vi "UserTable.vi"(8 "error in (no error)":errorcluster, 11 "MemberTable.lvclass":refnum<class "MemberTable.lvclass">) -> (0 "error out":errorcluster, 3 "MemberTable.lvclass":refnum<class "MemberTable.lvclass">)   [LabVIEW 2015, in "Member_Actor.lvlib"]
uses:
  Member_Actor.lvlib
  MemberTable/MemberTable.lvclass
  <vilib>/Utility/error.llb/Error Cluster From Error Code.vi
  <vilib>/ErrorRing/Error Ring.xnode
panel:
  in  "修改课程表":bool
  in  "课程表":cluster{"结束周":dbl, "起始周":dbl, "课程名称":string}[][](array[cluster])
  in  "Stop":bool
  # "—"
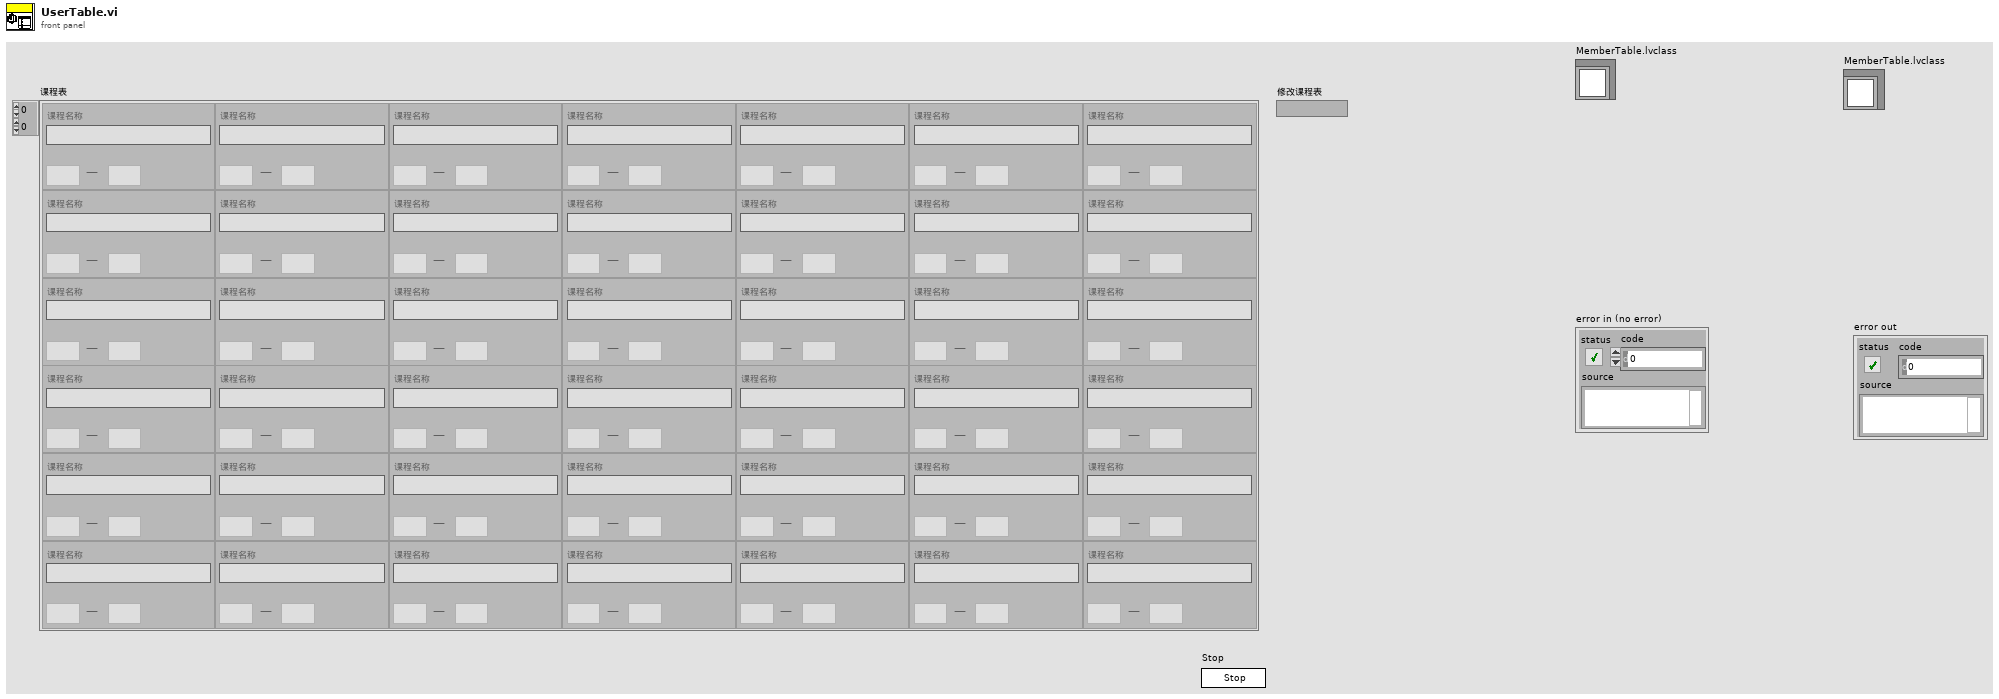
[diagram p1: front panel]
types:
  T1 = enum32{"Invalid", "Standard", "Closed", "Hidden", "Minimized", "Maximized"}
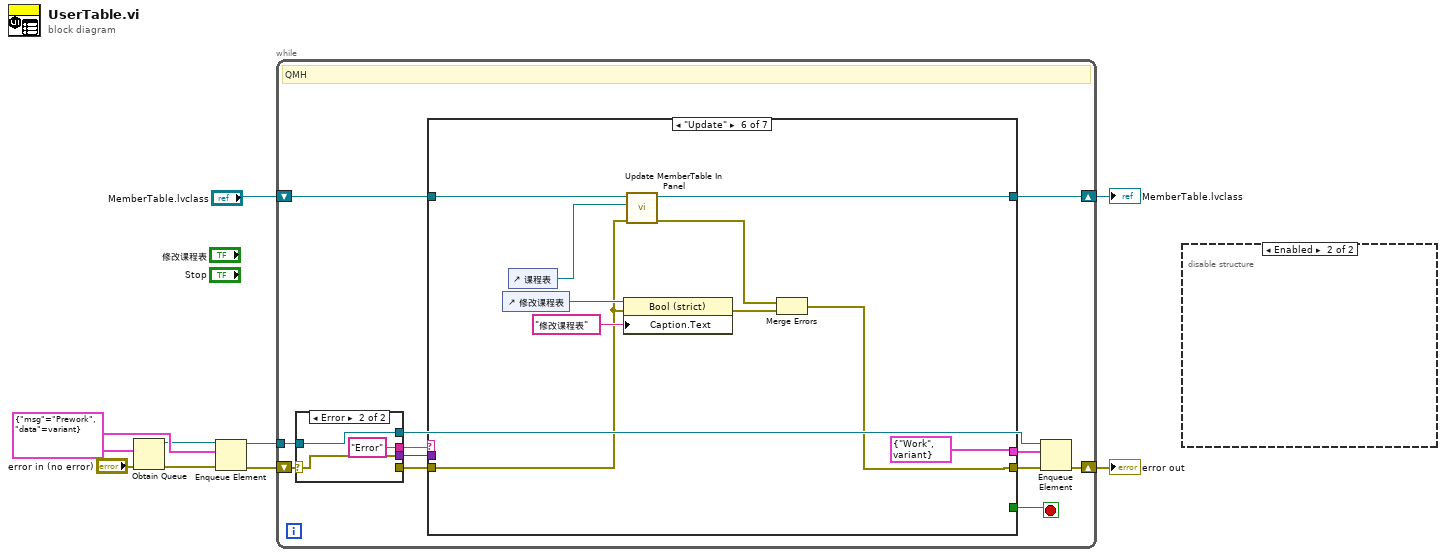
[diagram p0: block diagram]
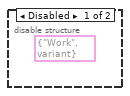
[diagram p2: hidden frame]
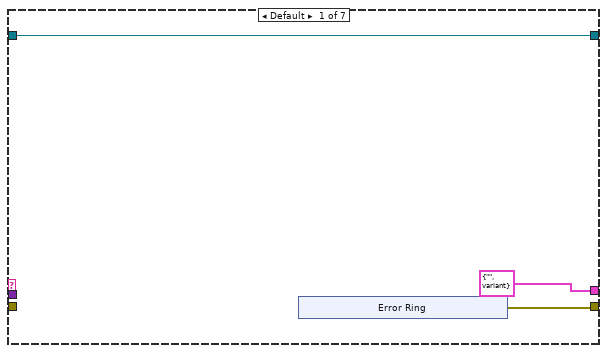
[diagram p3: hidden frame]
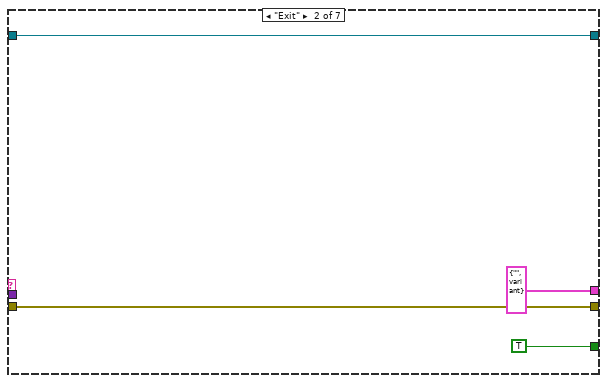
[diagram p4: hidden frame]
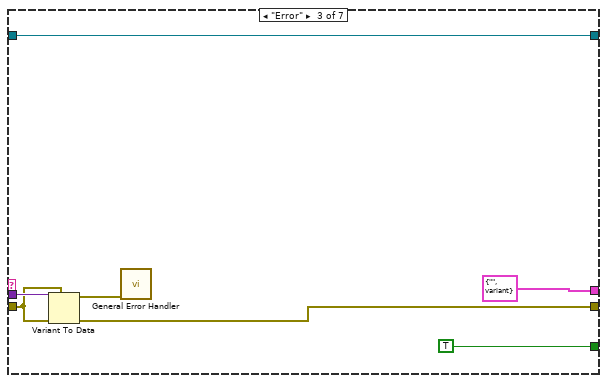
[diagram p5: hidden frame]
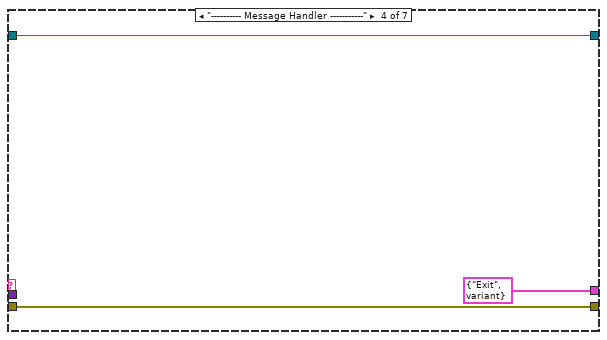
[diagram p6: hidden frame]
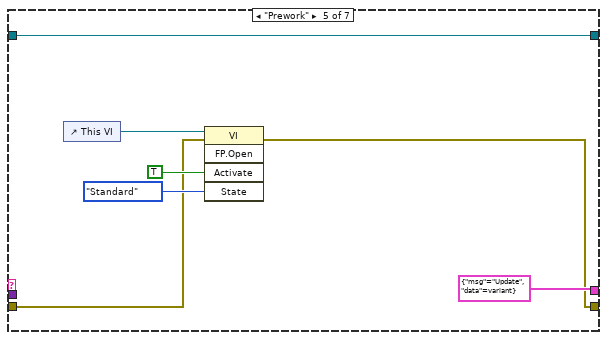
[diagram p7: hidden frame]
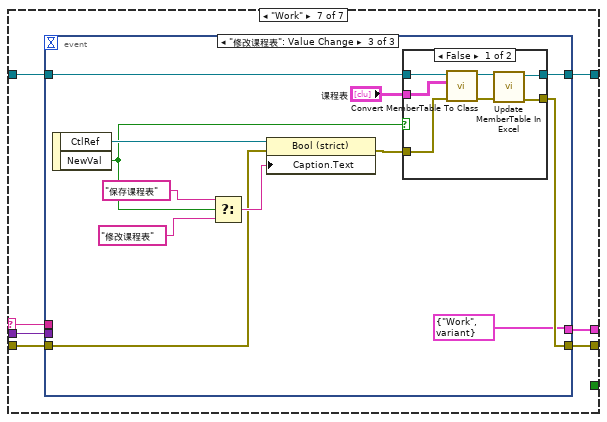
[diagram p8: hidden frame]
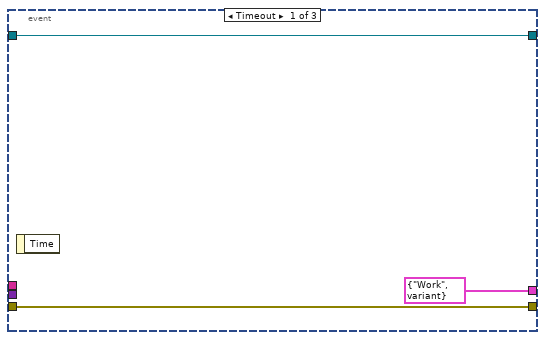
[diagram p9: hidden frame]
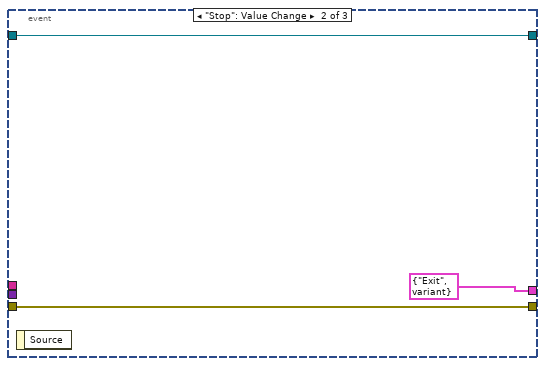
[diagram p10: hidden frame]
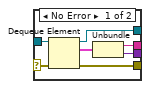
[diagram p12: hidden frame]
diagram:
  w7 = cluster{"msg":string, "data":variant} {"msg"="Prework", "data"=variant}
  n1 = Obtain Queue(element data type=w7, error in (no error)="error in (no error)") -> (queue out=w5:refnum<queue>, error out=w6:errorcluster)  [unwired: 3 in, 1 out]
  n2 = Enqueue Element(queue=w5, element=w7, error in (no error)=w6) -> (queue out=w8:refnum<queue>, error out=w9:errorcluster)  [unwired: 1 in, 1 out]
  n3 = while {
    tunnel: w8 -> [w20]
    shift-right: [w15] -> w2
    shift-left: w9 -> [w21]
    shift-right: [w10] -> w3
    shift-left: "MemberTable.lvclass" -> [w11]
    stop <- w12 stop-if-true
    # "QMH"
    n4 = case shown="Error" w21 {
      selector: w21 -> [w100 w104]
      tunnel: w20 -> [w101 w102]
      tunnel: [w99 _] -> w19
      tunnel: [w97 "Error" ("msg")] -> w18
      tunnel: [w96 w104] -> w17
      tunnel: [w95 w102] -> w14
      frame No Error {
        n5 = Dequeue Element(queue=w101, error in (no error)=w100) -> (queue out=w95:refnum<queue>, element=w98:cluster{"msg":string, "data":variant}, error out=w99:errorcluster)  [unwired: 1 in, 1 out]
        n6 = Unbundle(w98) -> ("msg"=w97:string, "data"=w96:variant)
      }
      frame Error {
      }
    }
    n7 = case shown="\"Update\"" w18 {
      selector: w18 -> [_ _ _ _ _ _ w65]
      tunnel: w19 -> [_ w33 w39 w43 w45 w55 w67]
      tunnel: w17 -> [_ _ w40 _ _ _ w66]
      tunnel: [w24 w33 w37 w43 w44 w52 w64] -> w16
      tunnel: [cluster{"msg":string, "data":variant} {"msg"="", "data"=variant} cluster{"msg":string, "data":variant} {"msg"="", "data"=variant} cluster{"msg":string, "data":variant} {"msg"="", "data"=variant} cluster{"msg":string, "data":variant} {"msg"="Exit", "data"=variant} cluster{"msg":string, "data":variant} {"msg"="Update", "data"=variant} cluster{"msg":string, "data":variant} {"msg"="Work", "data"=variant} w63] -> w13
      tunnel: [_ TRUE TRUE _ _ _ _] -> w12
      tunnel: w11 -> [w22 w30 w34 w41 w49 w59 w62]
      tunnel: [w22 w30 w34 w41 w49 w51 w61] -> w10
      frame Default {
        n8 = xnode "Error Ring"() -> ("error out"=w24:errorcluster)
      }
      frame "Exit" {
      }
      frame "Error" {
        n9 = Variant To Data(error in=w39, type=w39, Variant=w40) -> (data=w38:errorcluster, error out=w37:errorcluster)
        n10 = call <vilib>:"General Error Handler.vi"("error in (no error)"=w38) -> ()  [unwired: 10 in, 5 out]
      }
      frame "---------- Message Handler -----------" {
      }
      frame "Prework" {
        n11 = control-ref of="This VI"() -> (w48:refnum<vi>)
        n12 = invoke class="VI" method="FP.Open"(reference=w48, error in=w45, "Activate"=TRUE ("Activate?"), "State"=T1."Standard") -> (error out=w44:errorcluster)  [unwired: 1 in, 4 out]
      }
      frame "Update" {
        n13 = control-ref of="修改课程表"() -> (w57:refnum<vi>)
        n14 = control-ref of="课程表"() -> (w58:refnum<vi>)
        n15 = property class="Bool (strict)"(reference=w57, error in=w55, "Caption.Text"="修改课程表") -> (error out=w54:errorcluster)  [unwired: 1 out]
        n16 = call "Update MemberTable In Panel.vi"("error in (no error)"=w55, "课程表"=w58, "MemberTable in"=w59) -> ("error out"=w53:errorcluster, "MemberTable out"=w51:refnum<class "MemberTable.lvclass">)  [unwired: 7 in]
        n17 = Merge Errors(w53, w54) -> (w52:errorcluster)
      }
      frame "Work" {
        n18 = event shown="[2] \"修改课程表\": Value Change" {
          selector: _ -> [_ _ _]
          dyn-events: _ -> [_ _ _]
          timeout: _ -> [_ _ _]
          tunnel: w67 -> [w70 w73 w81]
          tunnel: w66 -> [_ _ _]
          tunnel: w65 -> [_ _ _]
          tunnel: [w70 w73 w75] -> w64
          tunnel: [cluster{"msg":string, "data":variant} {"msg"="Work", "data"=variant} cluster{"msg":string, "data":variant} {"msg"="Exit", "data"=variant} cluster{"msg":string, "data":variant} {"msg"="Work", "data"=variant}] -> w63
          tunnel: w62 -> [w68 w71 w79]
          tunnel: [w68 w71 w76] -> w61
          event Timeout {
            n19 = event-data() -> ()  [unwired: 1 in, 1 out]
          }
          event "Stop": Value Change {
            n20 = event-data() -> ()  [unwired: 1 in, 1 out]
          }
          event "修改课程表": Value Change {
            n21 = event-data() -> ("CtlRef"=w83:refnum<vi>, "NewVal"=w80:bool)  [unwired: 1 in]
            n22 = Select(t="保存课程表", s=w80, f="修改课程表") -> (s? t:f=w82:string)
            n23 = property class="Bool (strict)"(reference=w83, error in=w81, "Caption.Text"=w82) -> (error out=w77:errorcluster)  [unwired: 1 out]
            n24 = case shown="False" w80 {
              tunnel: w79 -> [w92 w94]
              tunnel: "课程表" -> [w91 _]
              tunnel: w77 -> [w90 w93]
              tunnel: [w87 w94] -> w76
              tunnel: [w86 w93] -> w75
              frame False {
                n25 = call "Convert MemberTable To Class.vi"("error in (no error)"=w90, "课程表"=w91, "MemberTable in"=w92) -> ("error out"=w88:errorcluster, "MemberTable out"=w89:refnum<class "MemberTable.lvclass">)  [unwired: 7 in]
                n26 = call "Update MemberTable In Excel.vi"("error in (no error)"=w88, "MemberTable in"=w89) -> ("error out"=w86:errorcluster, "MemberTable out"=w87:refnum<class "MemberTable.lvclass">)  [unwired: 8 in]
              }
              frame True {
              }
            }
          }
        }
      }
    }
    n27 = Enqueue Element(queue=w14, element=w13, error in (no error)=w16) -> (error out=w15:errorcluster)  [unwired: 1 in, 2 out]
  }
  "MemberTable.lvclass" <- w3
  "error out" <- w2
  n28 = disable-structure shown="Enabled" {
    frame Disabled {
      (unwired) cluster{"msg":string, "data":variant} {"msg"="Work", "data"=variant}
    }
    frame Enabled {
    }
  }
